vi "SequenceVI.vi"(7 "GUIRefArray":T1, 8 "error in":errorcluster, 10 "SlotEnable":enum16{"Enable", "Disable"}(ring)=enum."Disable", 11 "QueueIn":variant) -> (0 "error out":errorcluster)   [LabVIEW 2013]
uses:
  Ctl/States.ctl
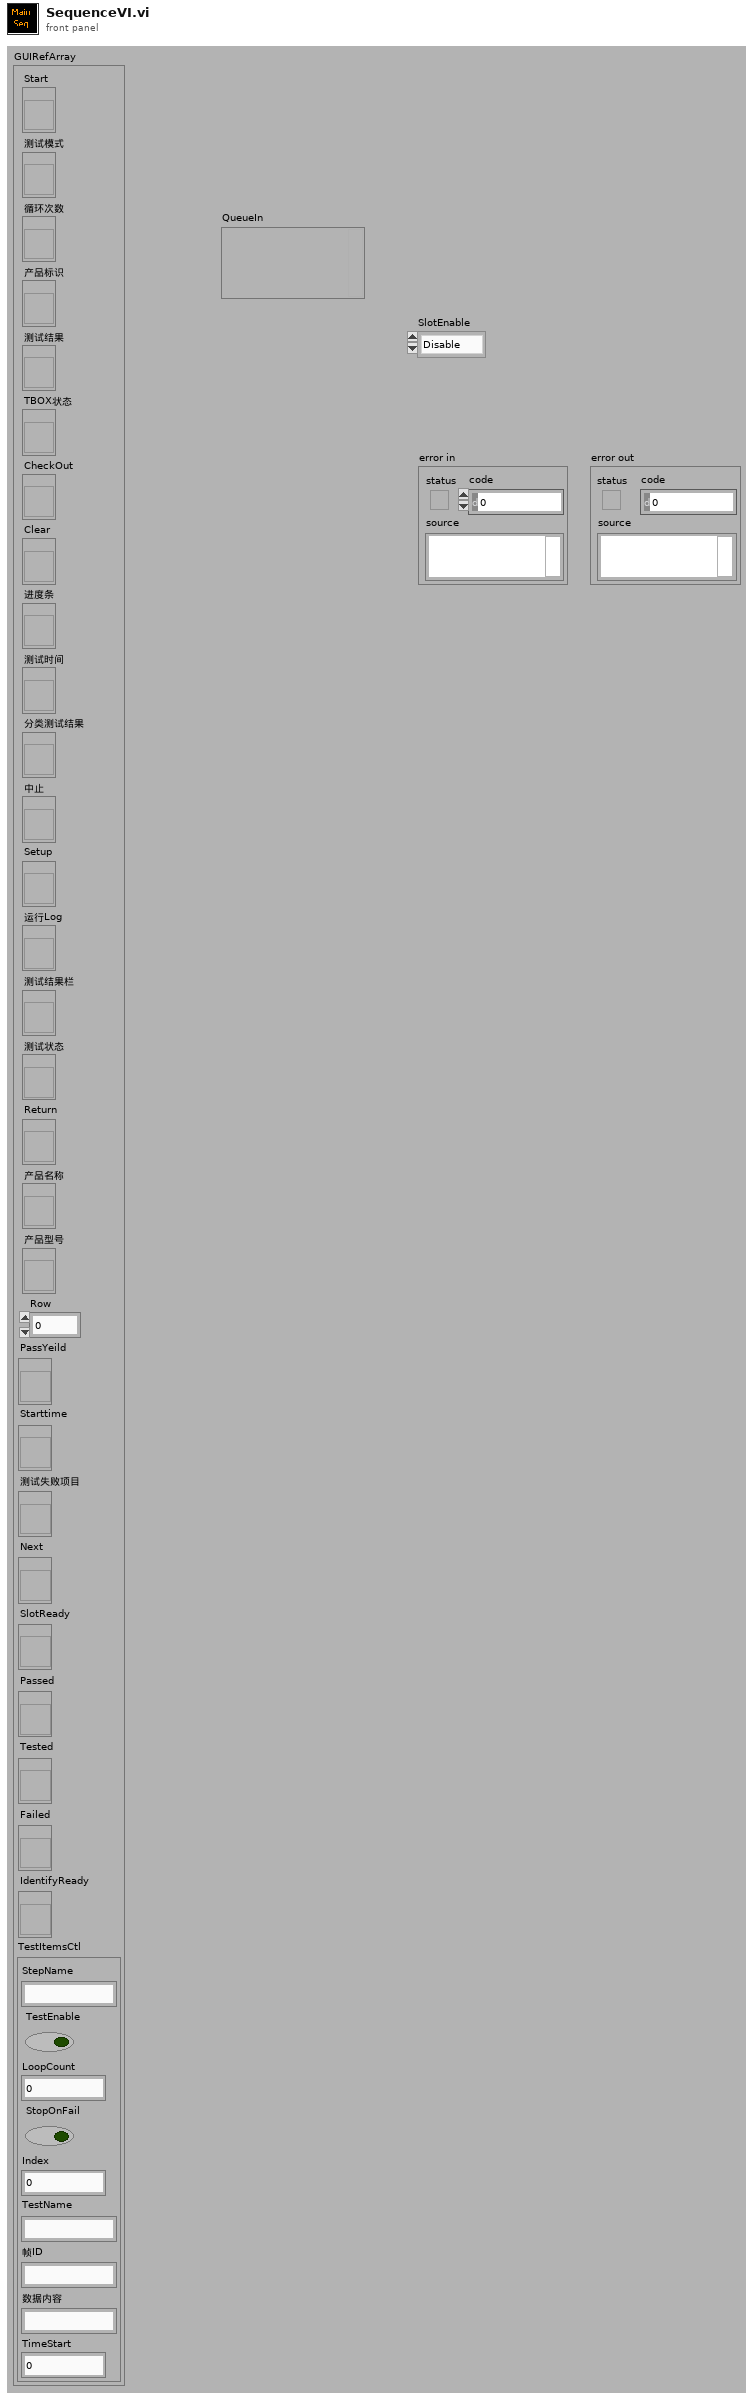
[diagram p1: front panel]
types:
  T1 = typedef "控件.ctl" = cluster{"Start":refnum<vi>, "测试模式":refnum<vi>, "循环次数":refnum<vi>, "产品标识":refnum<vi>, "测试结果":refnum<vi>, "TBOX状态":refnum<vi>, "CheckOut":refnum<vi>, "Clear":refnum<vi>, "进度条":refnum<vi>, "测试时间":refnum<vi>, "分类测试结果":refnum<vi>, "中止":refnum<vi>, "Setup":refnum<vi>, "运行Log":refnum<vi>, "测试结果栏":refnum<vi>, "测试状态":refnum<vi>, "Return":refnum<vi>, "产品名称":refnum<vi>, "产品型号":refnum<vi>, "Row":i32, "PassYeild":refnum<vi>, "Starttime":refnum<vi>, "测试失败项目":refnum<vi>, "Next":refnum<vi>, "SlotReady":refnum<vi>, "Passed":refnum<vi>, "Tested":refnum<vi>, "Failed":refnum<vi>, "IdentifyReady":refnum<vi>, "TestItemsCtl":cluster{"StepName":string, "TestEnable":bool, "LoopCount":u32, "StopOnFail":bool, "Index":u32, "TestName":string, "帧ID":string, "数据内容":string, "TimeStart":u32}}
  T2 = typedef "States.ctl" = enum16{"Init", "PreUUT", "Idle", "SetUp", "TestSequence", "PostUUT", "StopTest", "Debug Mode", "Selection Mode", "Loop Mode", "Error", "Wait"}
  T3 = enum16{"Production Mode", "Selection Mode", "Debug Mode", "Loop Mode"}
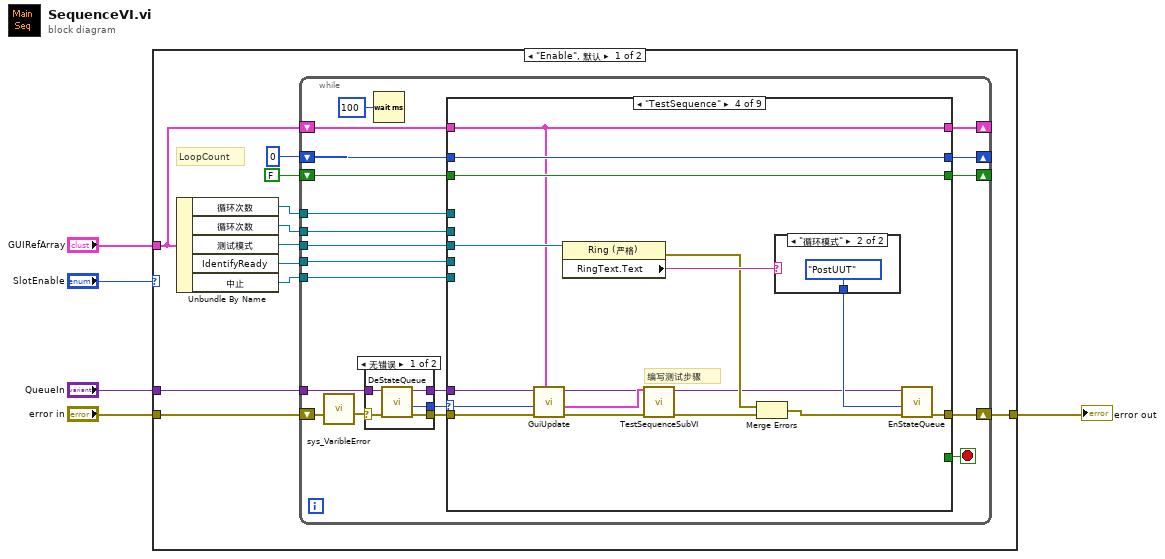
[diagram p0: block diagram]
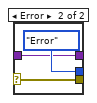
[diagram p2: hidden frame]
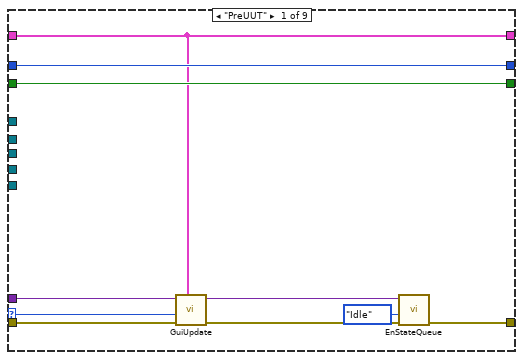
[diagram p3: hidden frame]
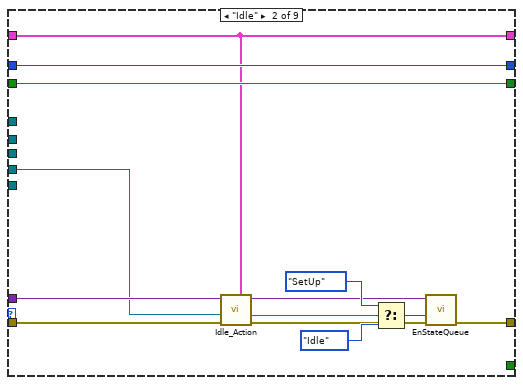
[diagram p4: hidden frame]
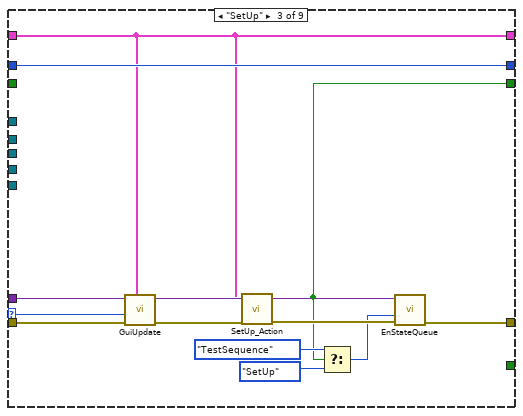
[diagram p5: hidden frame]
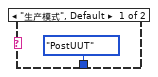
[diagram p6: hidden frame]
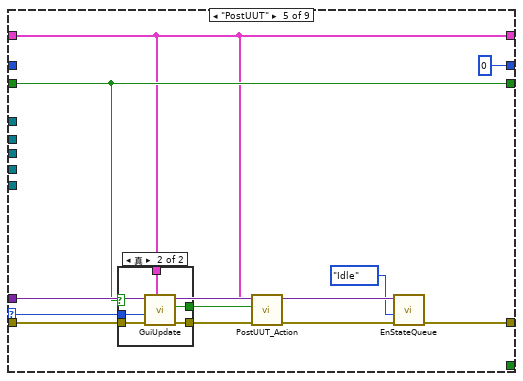
[diagram p7: hidden frame]
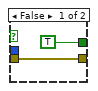
[diagram p8: hidden frame]
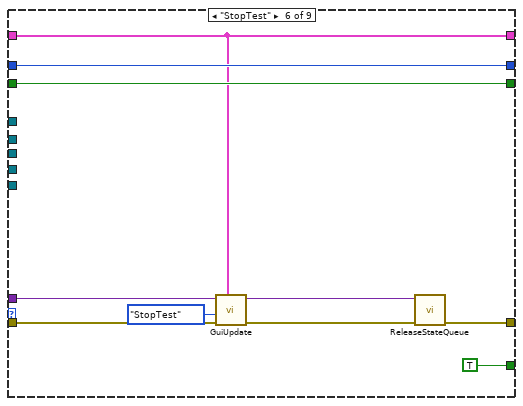
[diagram p9: hidden frame]
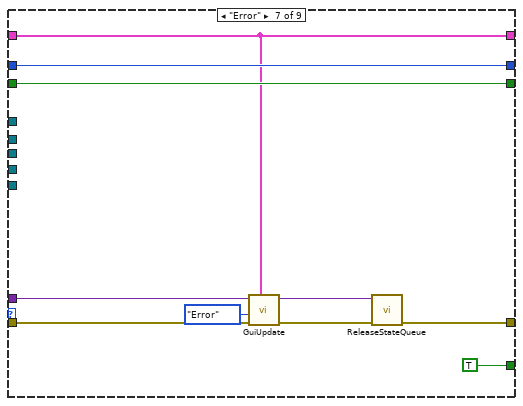
[diagram p10: hidden frame]
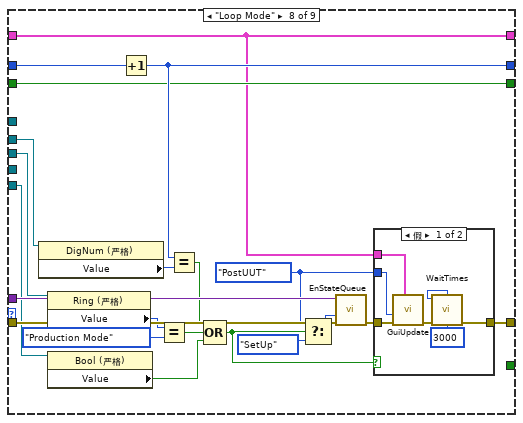
[diagram p11: hidden frame]
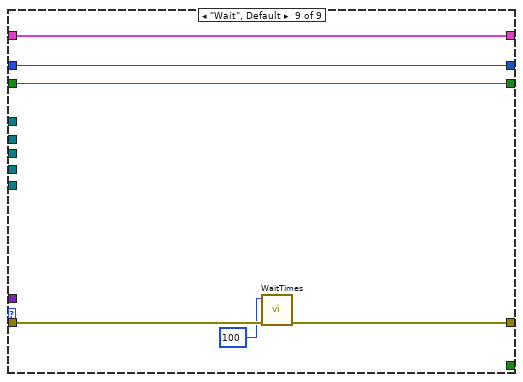
[diagram p13: hidden frame]
diagram:
  n1 = case shown="\"Enable\", 默认" "SlotEnable" {
    tunnel: "error in" -> [w12 w165]
    tunnel: [w11 w165] -> w3
    tunnel: "GUIRefArray" -> [w7 _]
    tunnel: "QueueIn" -> [w6 _]
    frame "Enable", Default {
      # "LoopCount"
      n2 = Unbundle By Name(w7) -> ("循环次数"=w15:refnum<vi>, "循环次数"=w13:refnum<vi>, "测试模式"=w14:refnum<vi>, "IdentifyReady"=w9:refnum<vi>, "中止"=w8:refnum<vi>)
      n3 = while {
        shift-right: [w33] -> w11
        shift-left: w12 -> [w18]
        tunnel: w6 -> [w34]
        shift-right: [w29] -> _
        shift-left: w7 -> [w30]
        shift-right: [w27] -> _
        shift-left: 0 -> [w28]
        tunnel: w14 -> [w26]
        tunnel: w15 -> [w25]
        tunnel: w13 -> [w24]
        shift-right: [w23] -> _
        shift-left: FALSE ("ScanSNOK") -> [w22]
        tunnel: w9 -> [w21]
        tunnel: w8 -> [w19]
        stop <- w35 stop-if-true
        n4 = call "sys_VaribleError.vi"("ErrorIn"=w18) -> ("ErrorOut"=w17:errorcluster)  [unwired: 10 in]
        n5 = case shown="无错误" w17 {
          selector: w17 -> [w41 w42]
          tunnel: [w40 w43] -> w36
          tunnel: [w39 w42] -> w31
          tunnel: [w37 States."Error" ("States")] -> w32
          tunnel: w34 -> [w38 w43]
          frame No Error {
            n6 = call "DeStateQueue.vi"("error in"=w41, "QueueIn"=w38) -> ("error out"=w39:errorcluster, "State"=w37:T2, "QueueOut"=w40:variant)  [unwired: 7 in]
          }
          frame Error {
          }
        }
        n7 = Wait (ms)(milliseconds to wait=u32 100 ("等待时间（毫秒）")) -> ()  [unwired: 1 out]
        n8 = case shown="\"TestSequence\"" w32 {
          selector: w32 -> [w51 _ w74 w89 w101 _ _ _ _]
          tunnel: w36 -> [w48 w64 w77 w78 w105 w121 w130 w151 _]
          tunnel: w31 -> [w53 w58 w75 w90 w102 w117 w126 w144 w164]
          tunnel: [_ _ _ _ _ TRUE TRUE _ _] -> w35
          tunnel: [w49 w62 w76 w92 w103 w118 w127 w145 w163] -> w33
          tunnel: w30 -> [w45 w54 w66 w83 w95 w114 w122 w133 w162]
          tunnel: [w45 w54 w66 w83 w95 w114 w122 w133 w162] -> w29
          tunnel: w28 -> [w52 w60 w73 w86 _ w119 w128 w150 w161]
          tunnel: [w52 w60 w73 w86 0 w119 w128 w148 w161] -> w27
          tunnel: w26 -> [_ _ _ w85 _ _ _ w140 _]
          tunnel: w25 -> [_ _ _ _ _ _ _ _ _]
          tunnel: w24 -> [_ _ _ _ _ _ _ w141 _]
          tunnel: [w46 w56 w67 w84 w97 w115 w124 w139 w160] -> w23
          tunnel: w22 -> [w46 w56 _ w84 w97 w115 w124 w139 w160]
          tunnel: w21 -> [_ w55 _ _ _ _ _ _ _]
          tunnel: w19 -> [_ _ _ _ _ _ _ w138 _]
          frame "PreUUT" {
            n9 = call "GuiUpdate.vi"("GuiRef"=w45, "error in"=w53, "States"=w51) -> ("error out"=w50:errorcluster)  [unwired: 2 in, 6 out]
            n10 = call "EnStateQueue.vi"("error in"=w50, "States"=States."Idle", "QueueIn"=w48) -> ("error out"=w49:errorcluster)  [unwired: 7 in, 1 out]
          }
          frame "Idle" {
            n11 = call "Idle_Action.vi"("GuiRef"=w54, "error in"=w58, "IdentifyReady"=w55) -> ("error out"=w59:errorcluster, "SlotReady"=w57:bool)  [unwired: 7 in]
            n12 = Select(t=States."SetUp" ("EnumOut"), s=w57, f=States."Idle" ("States")) -> (s? t:f=w63:T2)
            n13 = call "EnStateQueue.vi"("error in"=w59, "States"=w63, "QueueIn"=w64) -> ("error out"=w62:errorcluster)  [unwired: 7 in, 1 out]
          }
          frame "SetUp" {
            n14 = call "GuiUpdate.vi"("GuiRef"=w66, "error in"=w75, "States"=w74) -> ("error out"=w72:errorcluster)  [unwired: 2 in, 6 out]
            n15 = call "SetUp_Action.vi"("error in"=w72, "GuiRef"=w66) -> ("error out"=w71:errorcluster, "ScanSNOK"=w67:bool)  [unwired: 8 in]
            n16 = Select(t=States."TestSequence" ("States"), s=w67, f=States."SetUp" ("States")) -> (s? t:f=w69:T2)
            n17 = call "EnStateQueue.vi"("error in"=w71, "States"=w69, "QueueIn"=w77) -> ("error out"=w76:errorcluster)  [unwired: 7 in, 1 out]
          }
          frame "TestSequence" {
            # "编写测试步骤"
            n18 = call "GuiUpdate.vi"("GuiRef"=w83, "error in"=w90, "States"=w89) -> ("error out"=w91:errorcluster, "GuiRefOut"=w79:T1)  [unwired: 2 in, 5 out]
            n19 = property class="Ring (严格)"(reference=w85) -> (error out=w82:errorcluster, "RingText.Text"=w88:string)  [unwired: 1 in, 1 out]
            n20 = call "TestSequenceSubVI.vi"("GuiRef"=w79, "errorin"=w91) -> ("errorout"=w81:errorcluster)  [unwired: 13 in]
            n21 = Merge Errors(w82, w81) -> (w80:errorcluster)
            n22 = case shown="\"循环模式\"" w88 {
              tunnel: [States."PostUUT" ("States") States."PostUUT" ("States")] -> w87
              frame "生产模式", Default {
              }
              frame "循环模式" {
              }
            }
            n23 = call "EnStateQueue.vi"("error in"=w80, "States"=w87, "QueueIn"=w78) -> ("error out"=w92:errorcluster)  [unwired: 7 in, 1 out]
          }
          frame "PostUUT" {
            n24 = case shown="真" w97 {
              tunnel: w102 -> [w107 w112]
              tunnel: w101 -> [_ w111]
              tunnel: [w107 w110] -> w100
              tunnel: [TRUE ("PASS/FAIL") w108] -> w98
              tunnel: w95 -> [_ w109]
              frame False {
              }
              frame True {
                n25 = call "GuiUpdate.vi"("GuiRef"=w109, "error in"=w112, "States"=w111) -> ("error out"=w110:errorcluster, "PASS/FAIL"=w108:bool)  [unwired: 2 in, 5 out]
              }
            }
            n26 = call "PostUUT_Action.vi"("error in"=w100, "TestResult"=w98, "GuiRef"=w95) -> ("error out"=w99:errorcluster)  [unwired: 8 in]
            n27 = call "EnStateQueue.vi"("error in"=w99, "States"=States."Idle", "QueueIn"=w105) -> ("error out"=w103:errorcluster)  [unwired: 7 in, 1 out]
          }
          frame "StopTest" {
            n28 = call "GuiUpdate.vi"("GuiRef"=w114, "error in"=w117, "States"=States."StopTest") -> ("error out"=w113:errorcluster)  [unwired: 2 in, 6 out]
            n29 = call "ReleaseStateQueue.vi"("error in"=w113, "QueueIn"=w121) -> ("error out"=w118:errorcluster)  [unwired: 9 in]
          }
          frame "Error" {
            n30 = call "GuiUpdate.vi"("GuiRef"=w122, "error in"=w126, "States"=States."Error") -> ("error out"=w123:errorcluster)  [unwired: 2 in, 6 out]
            n31 = call "ReleaseStateQueue.vi"("error in"=w123, "QueueIn"=w130) -> ("error out"=w127:errorcluster)  [unwired: 9 in]
          }
          frame "Loop Mode" {
            w131 = States."PostUUT" ("States")
            n32 = property class="DigNum (严格)"(reference=w141) -> ("Value"=w149:u32)  [unwired: 1 in, 2 out]
            n33 = property class="Ring (严格)"(reference=w140) -> ("Value"=w143:u16)  [unwired: 1 in, 2 out]
            n34 = property class="Bool (严格)"(reference=w138) -> ("Value"=w135:bool)  [unwired: 1 in, 2 out]
            n35 = Increment(x=w150) -> (x+1=w148:i32)
            n36 = Equal?(x=w143, y=T3."Production Mode") -> (x = y?=w134:bool)
            n37 = Equal?(x=w148, y=w149) -> (x = y?=w136:bool)
            n38 = Compound Arithmetic op=OR(w136, w134, w135) -> (w137:bool)
            n39 = Select(t=w131, s=w137, f=States."SetUp" ("States")) -> (s? t:f=w146:T2)
            n40 = call "EnStateQueue.vi"("error in"=w144, "States"=w146, "QueueIn"=w151) -> ("error out"=w132:errorcluster)  [unwired: 7 in, 1 out]
            n41 = case shown="假" w137 {
              tunnel: w132 -> [w156 w158]
              tunnel: [w155 w158] -> w145
              tunnel: w133 -> [w153 _]
              tunnel: w131 -> [w154 _]
              frame False {
                n42 = call "GuiUpdate.vi"("GuiRef"=w153, "error in"=w156, "States"=w154) -> ("error out"=w157:errorcluster)  [unwired: 2 in, 6 out]
                n43 = call "WaitTimes.vi"("error in (no error)"=w157, "WaitTimes"=u32 3000) -> ("error out"=w155:errorcluster)  [unwired: 9 in]
              }
              frame True {
              }
            }
          }
          frame "Wait", Default {
            n44 = call "WaitTimes.vi"("error in (no error)"=w164, "WaitTimes"=u32 100) -> ("error out"=w163:errorcluster)  [unwired: 1 in, 8 out]
          }
        }
      }
    }
    frame "Disable" {
    }
  }
  "error out" <- w3
